vi "RT_Rotation_Integration (SubVI).vi"(0 "W(i) [rad/s] in":dbl[](array[numeric]), 1 "W_b(i) [rad/s]":dbl[](array[numeric]), 2 "ang_acc [rad/s^2]":dbl[](array[numeric]), 3 "D_NB":dbl[][](array[numeric]), 4 "q(i) in":dbl[](array[numeric]), 7 "dt":dbl, 9 "dt*0.5":dbl) -> (14 "W(i+1)":dbl[](array[numeric]), 16 "W_b(i+1) [rad/s]":dbl[](array[numeric]), 17 "q(i+1)":dbl[](array[numeric]), 19 "angles [rad]":dbl[](array[numeric]))   [LabVIEW 2017]
uses:
  <vilib>/Analysis/_algsub.llb/Vector Norm Type.ctl
  <vilib>/Analysis/coordinate.llb/Euler Rotation Order.ctl
  <vilib>/Analysis/baseanly.llb/Real A x B.vi
  <vilib>/Analysis/_algsub.llb/Real Vector Norm.vi
  <vilib>/Analysis/Matrix/Numeric/Conversions/Array To Matrix - RA.vi
  <vilib>/Analysis/Matrix/Numeric/Conversions/Array To Matrix - RA2.vi
  <vilib>/Analysis/Matrix/Numeric/Conversions/Matrix To Array - RM.vi
  <vilib>/Analysis/Matrix/NI_Matrix.lvlib
  <vilib>/Analysis/NI_AALBase.lvlib
  <vilib>/Analysis/NI_AALPro.lvlib
panel:
  out "Exp_Omega_k_T":dbl[][](array[numeric])
  out "S":dbl[][](array[numeric])
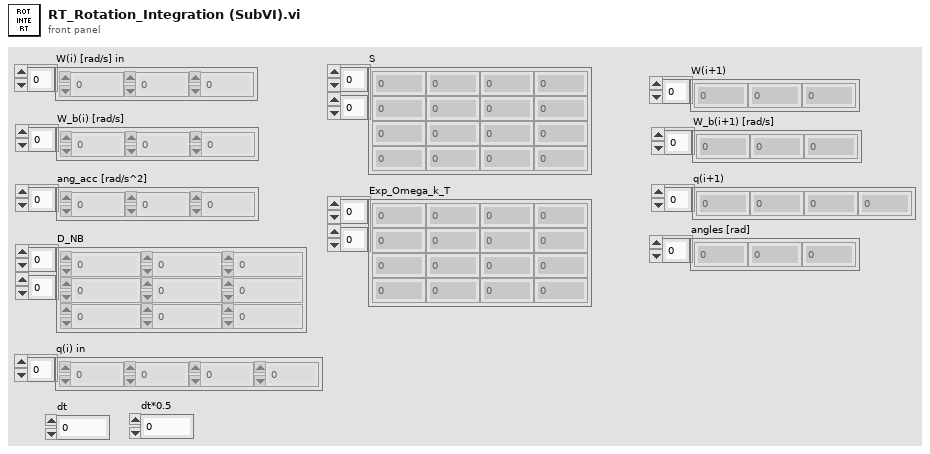
[diagram p1: front panel]
types:
  T1 = typedef "NI_AALPro.lvlib/Euler Rotation Order.ctl" = u16
  T2 = typedef "NI_AALPro.lvlib/Vector Norm Type.ctl" = u16
  T3 = typedef "NI_Matrix.lvlib/RealMatrix.ctl" = dbl[][]
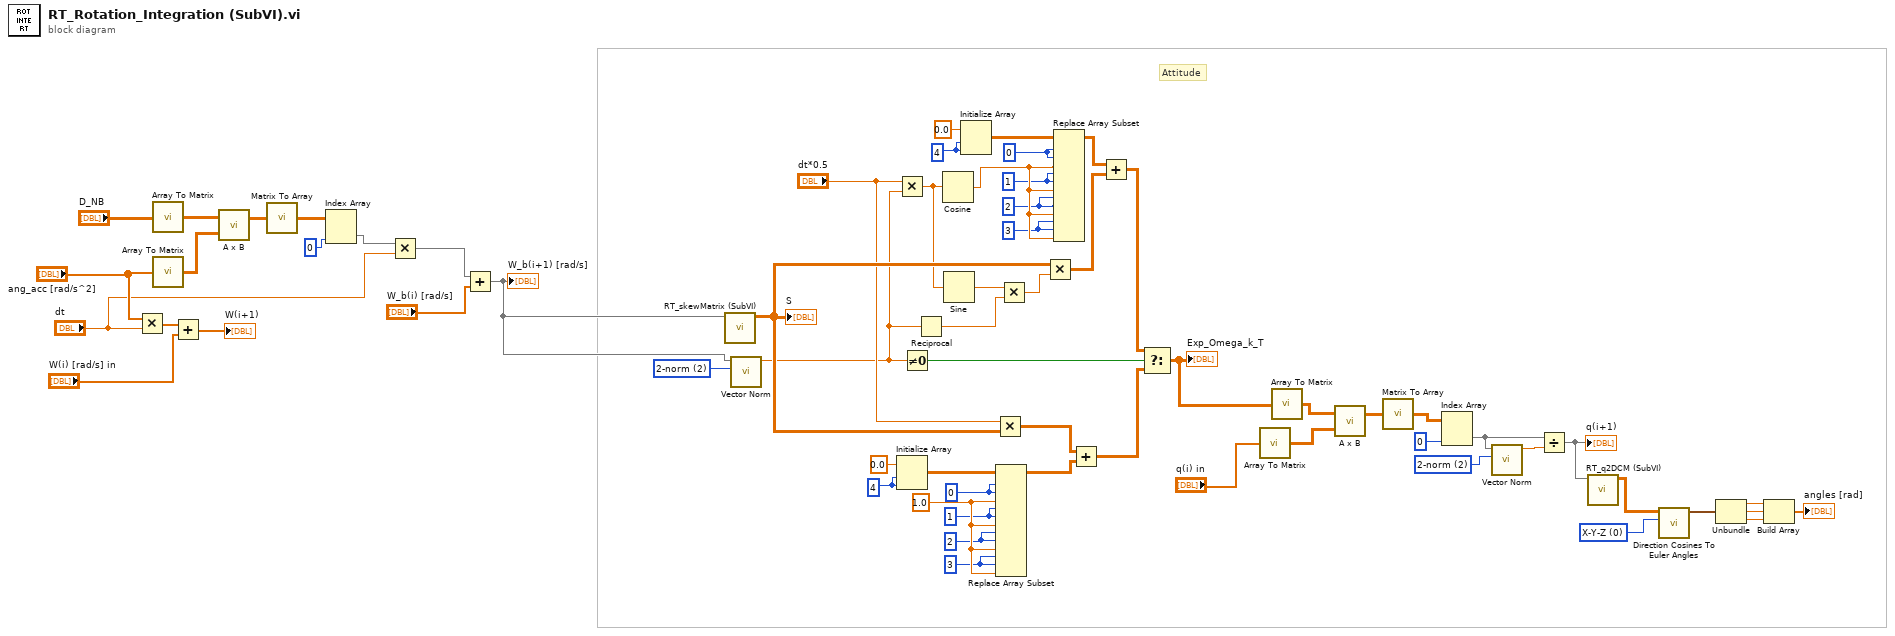
[diagram p0: block diagram]
diagram:
  w9 = T1 0 items=["X-Y-Z", "X-Z-Y", "Y-X-Z", "Y-Z-X", "Z-X-Y", "Z-Y-X", "X-Y-X", "X-Z-X", "Y-X-Y", "Y-Z-Y", "Z-X-Z", "Z-Y-Z"] ("rotation order")
  w60 = T2 2 items=["1-norm"=1, "2-norm"=2, "Inf-norm"=3, "-Inf-norm"=4, "User Defined"=5] ("norm type")
  w48 = 1.0 ("new element/subarray")
  w43 = 3 ("disabled index (row)")
  w42 = 2 ("disabled index (row)")
  w41 = 1 ("disabled index (row)")
  w44 = 0 ("disabled index (row)")
  w47 = 4 ("dimension size")
  w36 = 3 ("disabled index (row)")
  w37 = 2 ("disabled index (row)")
  w38 = 1 ("disabled index (row)")
  w35 = 0 ("disabled index (row)")
  w25 = 4 ("dimension size")
  w23 = T2 2 items=["1-norm"=1, "2-norm"=2, "Inf-norm"=3, "-Inf-norm"=4, "User Defined"=5] ("norm type")
  # "Attitude"
  n1 = Multiply(x="ang_acc [rad/s^2]", y="dt") -> (x*y=w63:dbl[])
  n2 = call-poly <vilib>:"Array To Matrix.vi"("Real 2D Array"="D_NB") -> ("Real Matrix"=w20:T3)
  n3 = call-poly <vilib>:"Array To Matrix.vi"("Real 1D Array"="ang_acc [rad/s^2]") -> ("Real Matrix (Column Vector)"=w19:T3)
  n4 = Add ("Add.vi")(x=w63, y="W(i) [rad/s] in") -> (x+y=→"W(i+1)":dbl[])
  n5 = call-poly <vilib>:"A x B.vi"("B"=w19, "A"=w20) -> ("A x B"=w17:T3)  [unwired: 1 out]
  n6 = call-poly <vilib>:"Matrix To Array.vi"("Real Matrix"=w17) -> ("Real 2D Array"=w18:dbl[][])
  n7 = Index Array(array=w18, index (col)=0 ("index (row)")) -> (element=w13:dbl[])  [unwired: 1 in]
  n8 = Multiply(x=w13, y="dt") -> (x*y=w11:dbl[])
  n9 = Add(x=w11, y="W_b(i) [rad/s]") -> (x+y=w1:dbl[])
  "W_b(i+1) [rad/s]" <- w1
  n10 = call "RT_skewMatrix (SubVI).vi"("vector"=w1) -> ("skew matrix"=w50:dbl[][])  [unwired: 10 in]
  "S" <- w50
  n11 = call-poly <vilib>:"Vector Norm.vi"("norm type"=w23, "Input Vector"=w1) -> ("norm"=w28:dbl)  [unwired: 8 in, 1 out]
  n12 = Multiply(x="dt*0.5", y=w28) -> (x*y=w27:dbl)
  n13 = Initialize Array(0.0 ("element"), w47, w47) -> (w45:dbl[][])
  n14 = Not Equal To 0?(x=w28) -> (x != 0?=w24:bool)
  n15 = Reciprocal(x=w28) -> (1/x=w30:dbl)
  n16 = Cosine(x=w27) -> (cos(x)=w39:dbl)
  n17 = Sine(x=w27) -> (sin(x)=w29:dbl)
  n18 = Initialize Array(0.0 ("element"), w25, w25) -> (w33:dbl[][])
  n19 = Multiply(x="dt*0.5", y=w50) -> (x*y=w51:dbl[][])
  n20 = Replace Array Subset(array=w45, new element #1=w48, index (row) #1=w44, index (col) #1=w44, new element #2=w48, index (row) #2=w41, index (col) #2=w41, new element #3=w48, index (row) #3=w42, index (col) #3=w42, new element #4=w48, index (row) #4=w43, index (col) #4=w43) -> (w52:dbl[][])
  n21 = Multiply(x=w29, y=w30) -> (x*y=w31:dbl)
  n22 = Multiply(x=w50, y=w31) -> (x*y=w32:dbl[][])
  n23 = Replace Array Subset(array=w33, new element #1=w39, index (row) #1=w35, index (col) #1=w35, new element #2=w39, index (row) #2=w38, index (col) #2=w38, new element #3=w39, index (row) #3=w37, index (col) #3=w37, new element #4=w39, index (row) #4=w36, index (col) #4=w36) -> (w34:dbl[][])
  n24 = Add ("Add.vi")(x=w51, y=w52) -> (x+y=w53:dbl[][])
  n25 = Add ("Add.vi")(x=w34, y=w32) -> (x+y=w40:dbl[][])
  n26 = Select(t=w40, s=w24, f=w53) -> (s? t:f=w59:dbl[][])
  "Exp_Omega_k_T" <- w59
  n27 = call-poly <vilib>:"Array To Matrix.vi"("Real 1D Array"="q(i) in") -> ("Real Matrix (Column Vector)"=w57:T3)
  n28 = call-poly <vilib>:"Array To Matrix.vi"("Real 2D Array"=w59) -> ("Real Matrix"=w58:T3)
  n29 = call-poly <vilib>:"A x B.vi"("B"=w57, "A"=w58) -> ("A x B"=w55:T3)  [unwired: 1 out]
  n30 = call-poly <vilib>:"Matrix To Array.vi"("Real Matrix"=w55) -> ("Real 2D Array"=w56:dbl[][])
  n31 = Index Array(array=w56, index (col)=0 ("index (row)")) -> (element=w62:dbl[])  [unwired: 1 in]
  n32 = call-poly <vilib>:"Vector Norm.vi"("norm type"=w60, "Input Vector"=w62) -> ("norm"=w61:dbl)  [unwired: 8 in, 1 out]
  n33 = Divide(x=w62, y=w61) -> (x/y=w4:dbl[])
  "q(i+1)" <- w4
  n34 = call "RT_q2DCM (SubVI).vi"("Quaternion"=w4) -> ("DCM"=w3:dbl[][])  [unwired: 10 in]
  n35 = call <vilib>:"Direction Cosines To Euler Angles.vi"("rotation order"=w9, "Direction Cosines"=w3) -> ("Euler Angles"=w6:cluster{"phi":dbl, "theta":dbl, "psi":dbl})  [unwired: 8 in, 1 out]
  n36 = Unbundle(w6) -> ("phi"=w8:dbl, "theta"=w7:dbl, "psi"=w5:dbl)
  n37 = Build Array(w8, w7, w5) -> (→"angles [rad]":dbl[])
